vi "Create Variables for Picture Rings.vi"(8 "error in (no error)":errorcluster, 11 "Web FP In":refnum<class "Web Front Panel.lvclass">) -> (0 "error out":errorcluster, 3 "Variables String":string)   [LabVIEW 2017, in "Front Panel Publisher.lvlib" / "Web Front Panel.lvclass"]
uses:
  Web Front Panel.lvclass
  Front Panel Publisher.lvlib
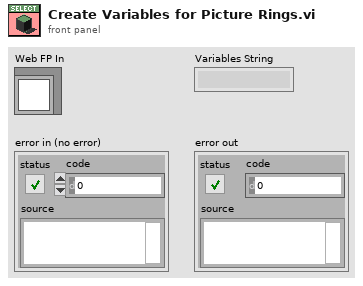
[diagram p1: front panel]
types:
  T1 = typedef "Front Panel Publisher.lvlib/Web Front Panel.lvclass/Object Attributes.ctl" = cluster{"VI Identifier":string, "VI Reference":refnum<vi>, "Controls":refnum<class "Object.lvclass">[], "Indicators":refnum<class "Object.lvclass">[], "Decorations":refnum<class "Object.lvclass">[], "VR With Previous Get":refnum<data-value>, "VR With Ring Images":refnum<data-value>}
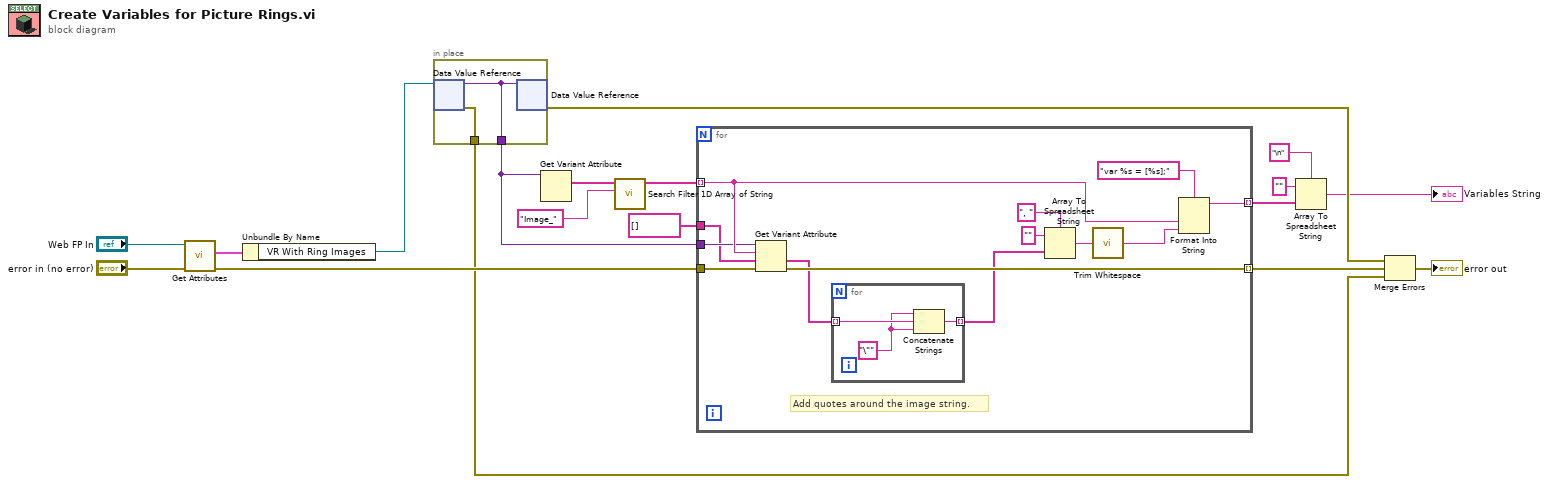
[diagram p0: block diagram]
diagram:
  n1 = call "Get Attributes.vi"("error in (no error)"="error in (no error)", "Web FP In"="Web FP In") -> ("error out"=w16:errorcluster, "Data"=w13:T1)  [unwired: 6 in, 2 out]
  n2 = Unbundle By Name(w13) -> ("VR With Ring Images"=w15:refnum<data-value>)
  n3 = in-place {
    in-place-border: [w20] -> w9
    in-place-border: [w19] -> w11
    n4 = in-place-dvr #1(w15) -> (w20:variant, w19:errorcluster)
    n5 = in-place-dvr #1(w20) -> (w10:errorcluster)  [unwired: 1 out]
  }
  n6 = Get Variant Attribute(Variant=w9) -> (names=w8:string[])  [unwired: 3 in, 3 out]
  n7 = call "Search Filter 1D Array of String.vi"("Search String"="Image_", "String Array to Search"=w8) -> ("Matching Elements"=w6:string[])  [unwired: 7 in, 2 out]
  n8 = for {
    tunnel: w9 -> [w26]
    tunnel: w6 -> [w27] mode=indexing
    tunnel: w16 -> [w24]
    tunnel: [w23] -> w17 mode=indexing
    tunnel: [w28] -> w5 mode=indexing
    tunnel: string[] [] -> [w25]
    # "Add quotes around the image string."
    n9 = Get Variant Attribute(Variant=w26, name=w27, default value (empty Variant)=w25, error in=w24) -> (value=w22:string[], error out=w23:errorcluster)  [unwired: 2 out]
    n10 = for {
      tunnel: w22 -> [w36] mode=indexing
      tunnel: [w34] -> w21 mode=indexing
      w35 = "\""
      n11 = Concatenate Strings(w35, w36, w35) -> (w34:string)
    }
    n12 = Array To Spreadsheet String(delimiter (Tab)=", ", array=w21, 3:"" ("format string")) -> (spreadsheet string=w30:string)
    n13 = call <vilib>:"Trim Whitespace.vi"("string"=w30) -> ("trimmed string"=w29:string)  [unwired: 1 in]
    n14 = Format Into String(format string="var %s = [%s];", w27, w29) -> (resulting string=w28:string)  [unwired: 2 in, 1 out]
  }
  n15 = Array To Spreadsheet String(delimiter (Tab)="\n", array=w5, 3:"" ("format string")) -> (spreadsheet string=→"Variables String":string)
  n16 = Merge Errors(w10, w17, w11) -> (→"error out":errorcluster)
